vi "Bridge.vi"() -> ()   [LabVIEW 2012]
panel:
  out "Kill":bool
  # "Update the project properties to point at your cRIO's IP and then run me."
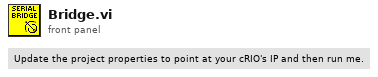
[diagram p1: front panel]
types:
  T1 = typedef "WPI_SerialPortRef.ctl" = cluster{"DevStatus":errorcluster, "Serial Port Name":refnum<visa-resource-name>}
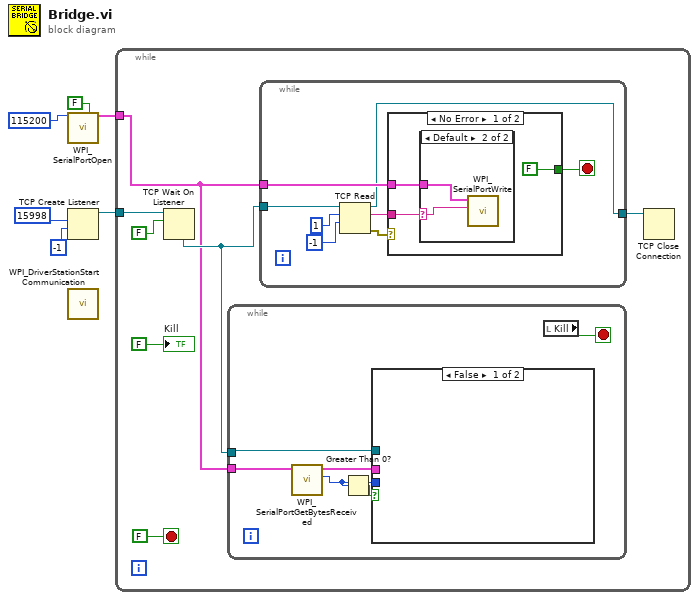
[diagram p0: block diagram]
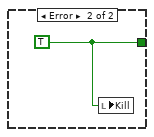
[diagram p3: hidden frame]
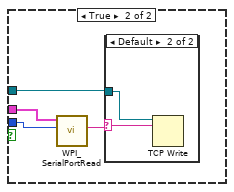
[diagram p4: hidden frame]
diagram:
  n1 = call <vilib>:"WPI_SerialPortOpen.vi"("Baud Rate"=u32 115200, "Enable Termination Char? (T)"=FALSE) -> ("SerialPortRef"=w4:T1)  [unwired: 12 in, 1 out]
  n2 = TCP Create Listener(9:-1 ("timeout ms (25000)"), 10:u16 15998 ("port")) -> (3:w2:refnum<k5>)  [unwired: 3 in, 2 out]
  n3 = call <vilib>:"WPI_DriverStationStart Communication.vi"() -> ()  [unwired: 12 in]
  n4 = while {
    tunnel: w4 -> [w7]
    tunnel: w2 -> [w13]
    stop <- FALSE stop-if-true
    n5 = TCP Wait On Listener(10:FALSE ("resolve remote address (T)"), 11:w13) -> (4:w11:refnum<k5>)  [unwired: 2 in, 4 out]
    n6 = while {
      tunnel: w7 -> [w31]
      tunnel: w11 -> [w33]
      stop <- w28 stop-if-true
      n7 = call <vilib>:"WPI_SerialPortGetBytesReceived.vi"("SerialPortRef"=w31) -> ("Bytes at Port"=w29:u32, "SerialPortRef"=w30:T1)  [unwired: 8 in, 1 out]
      n8 = Greater Than 0?(x=w29) -> (x > 0?=w32:bool)
      n9 = case shown="False" w32 {
        tunnel: w30 -> [_ w37]
        tunnel: w33 -> [_ w36]
        tunnel: w29 -> [_ w34]
        frame False {
        }
        frame True {
          n10 = call <vilib>:"WPI_SerialPortRead.vi"("Num Bytes to Read"=w34, "SerialPortRef"=w37) -> ("Buffer"=w35:string)  [unwired: 7 in, 2 out]
          n11 = case shown="Default" w35 {
            selector: w35 -> [_ w38]
            tunnel: w36 -> [_ w39]
            frame "" {
            }
            frame Default {
              n12 = TCP Write(connection ID=w39, data in=w38) -> ()  [unwired: 2 in, 3 out]
            }
          }
        }
      }
      n13 = local read "Kill"() -> (w28:bool)
    }
    n14 = while {
      tunnel: w11 -> [w21]
      tunnel: w7 -> [w19]
      tunnel: [w14] -> w9
      stop <- w15 stop-if-true
      n15 = TCP Read(connection ID=w21, bytes to read=1, 9:-1 ("timeout ms (25000)")) -> (connection ID out=w14:refnum<k5>, data out=w17:string, error out=w16:errorcluster)  [unwired: 2 in]
      n16 = case shown="No Error" w16 {
        tunnel: w19 -> [w24 _]
        tunnel: w17 -> [w23 _]
        tunnel: [FALSE w27] -> w15
        frame No Error {
          n17 = case shown="Default" w23 {
            selector: w23 -> [_ w25]
            tunnel: w24 -> [_ w26]
            frame "" {
            }
            frame Default {
              n18 = call <vilib>:"WPI_SerialPortWrite.vi"("Buffer"=w25, "SerialPortRef"=w26) -> ()  [unwired: 7 in, 3 out]
            }
          }
        }
        frame Error {
          w27 = TRUE
          n19 = local write "Kill"(w27) -> ()
        }
      }
    }
    n20 = TCP Close Connection(connection ID=w9) -> ()  [unwired: 2 in, 2 out]
    "Kill" <- FALSE ("Kill")
  }
